vi "zadanie1.vi"() -> ()   [LabVIEW 2012]
panel:
  out "Wykres zmiany V":cluster{i32, dbl}[](graph)
  # "trzeba tyklko poprawic opisy, podpisy i to co jest na dole wykresu"
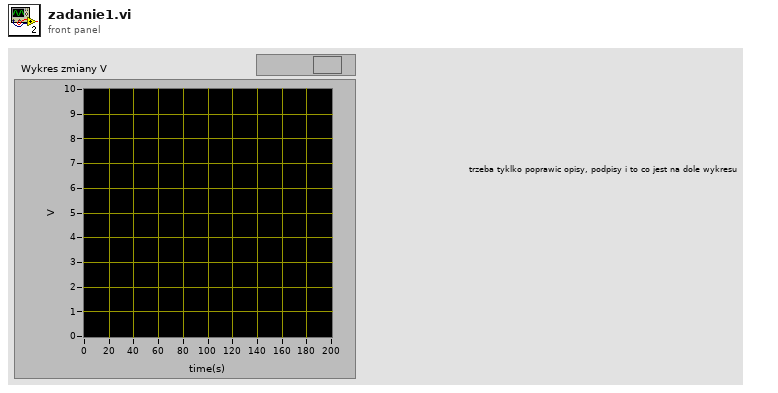
[diagram p1: front panel]
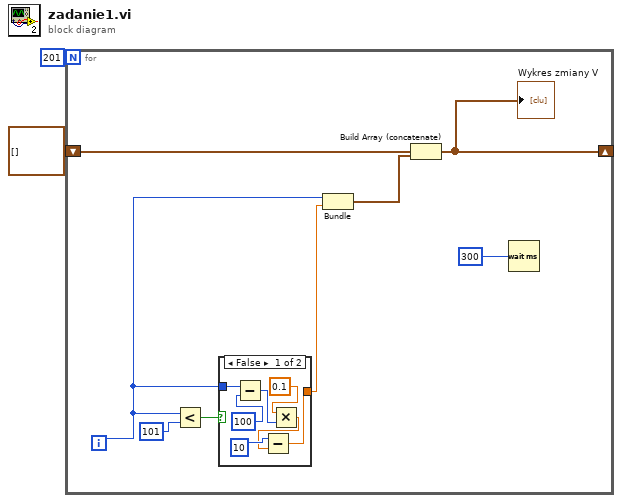
[diagram p0: block diagram]
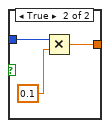
[diagram p2: hidden frame]
diagram:
  n1 = for {
    N: 201 -> [_]
    shift-right: [w8] -> _
    shift-left: cluster{i32, i32}[] [] -> [w7]
    i -> [w4]
    n2 = Less?(x=w4, y=101) -> (x < y?=w5:bool)
    n3 = case shown="False" w5 {
      tunnel: w4 -> [w17 w19]
      tunnel: [w11 w18] -> w6
      frame False {
        n4 = Subtract(x=w17, y=100) -> (x-y=w16:i32)
        n5 = Multiply(x=0.1, y=w16) -> (x*y=w12:dbl)
        n6 = Subtract(x=10, y=w12) -> (x-y=w11:dbl)
      }
      frame True {
        n7 = Multiply(x=w19, y=0.1) -> (x*y=w18:dbl)
      }
    }
    n8 = Bundle(w4, w6) -> (w9:cluster{i32, dbl})  [unwired: 1 in]
    n9 = Build Array (concatenate)(w7, w9) -> (w8:cluster{i32, dbl}[])
    "Wykres zmiany V" <- w8
    n10 = Wait (ms)(milliseconds to wait=300) -> ()  [unwired: 1 out]
  }
